vi "air.vi"() -> ()   [LabVIEW 2018]
panel:
  in  "Numeric":dbl
  in  "Numeric 2":dbl
  out "String 2":string
  out "String":string
  out "fan":dbl(slide) scale=0.0..10.0
  in  "stop 2":bool
  in  "temp-":bool
  in  "temp+":bool
  in  "stop":bool
  out "temp":dbl
  out "7 2":bool
  out "6 2":bool
  out "5 2":bool
  out "4 2":bool
  out "3 2":bool
  out "2 2":bool
  out "1 2":bool
  out "7":bool
  out "6":bool
  out "5":bool
  out "4":bool
  out "3":bool
  out "2":bool
  out "1":bool
  in  "TIMER":bool
  in  "Bio sleep":bool
  in  "Auto clean":bool
  in  "Turbo":bool
  in  "Mode":bool
  in  "swing":bool
  in  "on/off":bool
  in  "fan-":bool
  in  "fan+":bool
  # "TEMP"
  # "FAN"
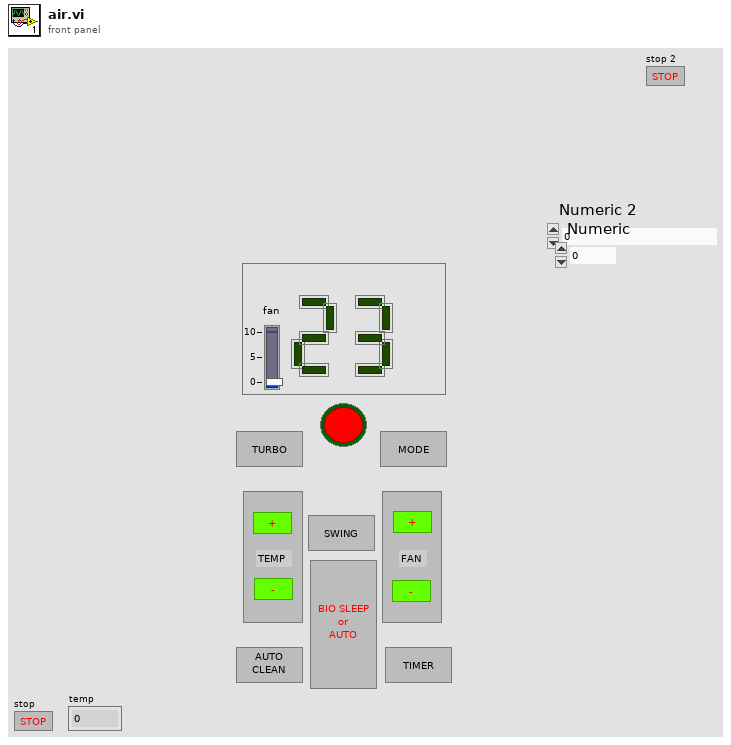
[diagram p1: front panel]
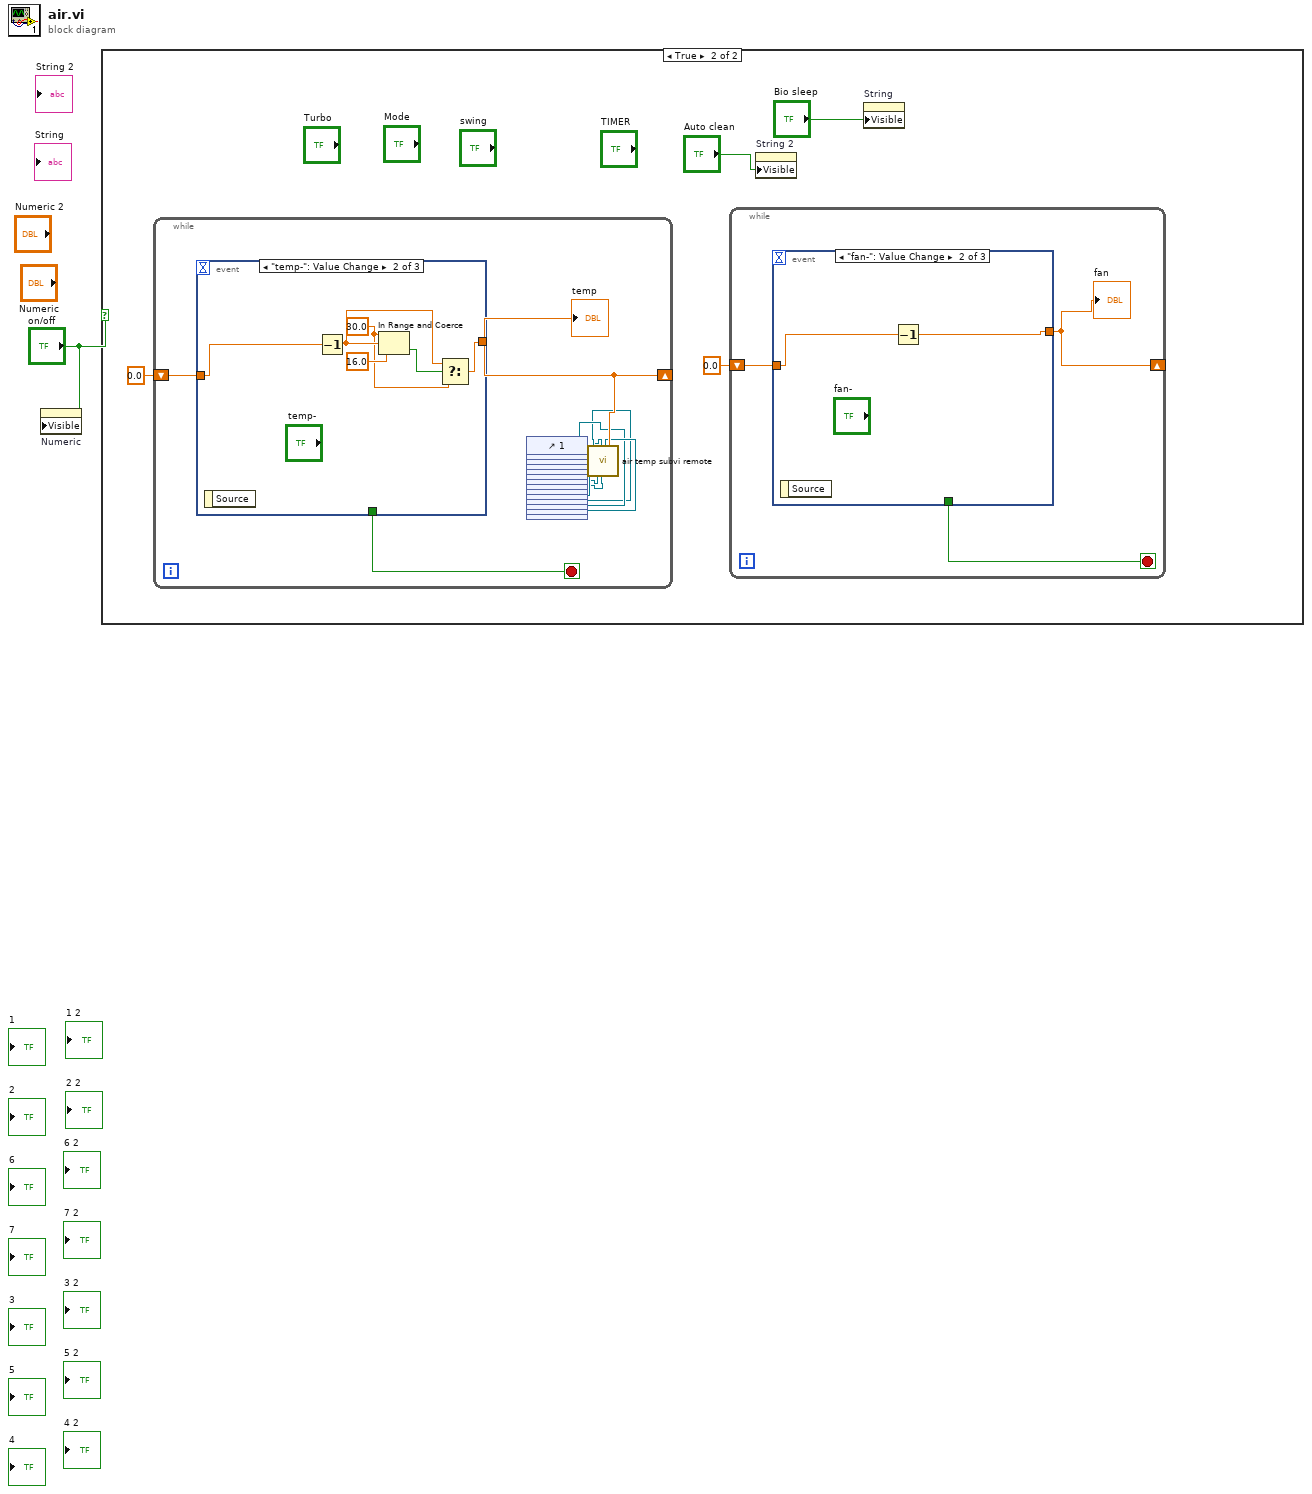
[diagram p0: block diagram]
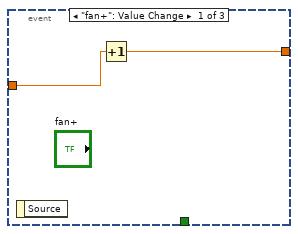
[diagram p3: hidden frame]
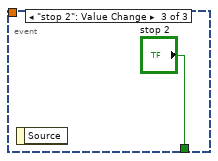
[diagram p4: hidden frame]
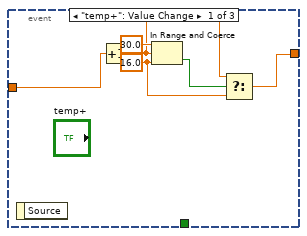
[diagram p5: hidden frame]
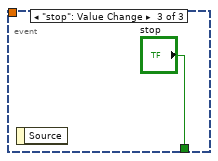
[diagram p6: hidden frame]
diagram:
  n1 = property on="Numeric" class="DigNum (strict)"("Visible"="on/off") -> ()  [unwired: 2 in, 2 out]
  n2 = case shown="True" "on/off" {
    frame False {
    }
    frame True {
      n3 = while {
        shift-right: [w28] -> _
        shift-left: 0.0 -> [w30]
        stop <- w29 stop-if-true
        n4 = event shown="[1] \"temp-\": Value Change" {
          selector: _ -> [_ _ _]
          dyn-events: _ -> [_ _ _]
          timeout: _ -> [_ _ _]
          tunnel: [w35 w37 _] -> w28
          tunnel: w30 -> [w36 w42 _]
          tunnel: [_ _ "stop"] -> w29
          event "temp+": Value Change {
            w31 = 16.0 ("lower limit")
            n5 = event-data() -> ()  [unwired: 1 in, 1 out]
            n6 = Increment(x=w36) -> (x+1=w32:dbl)
            n7 = In Range and Coerce(upper limit=30.0, x=w32, lower limit=w31) -> (In Range?=w33:bool)  [unwired: 1 out]
            n8 = Select(t=w32, s=w33, f=w31) -> (s? t:f=w35:dbl)
          }
          event "temp-": Value Change {
            w38 = 30.0 ("upper limit")
            n9 = event-data() -> ()  [unwired: 1 in, 1 out]
            n10 = Decrement(x=w42) -> (x-1=w39:dbl)
            n11 = In Range and Coerce(upper limit=w38, x=w39, lower limit=16.0) -> (In Range?=w41:bool)  [unwired: 1 out]
            n12 = Select(t=w39, s=w41, f=w38) -> (s? t:f=w37:dbl)
          }
          event "stop": Value Change {
            n13 = event-data() -> ()  [unwired: 1 in, 1 out]
          }
        }
        "temp" <- w28
        n14 = control-ref of="1"() -> (w14:refnum<vi>)
        n15 = control-ref of="2"() -> (w15:refnum<vi>)
        n16 = control-ref of="3"() -> (w16:refnum<vi>)
        n17 = control-ref of="4"() -> (w17:refnum<vi>)
        n18 = control-ref of="5"() -> (w18:refnum<vi>)
        n19 = control-ref of="6"() -> (w19:refnum<vi>)
        n20 = control-ref of="7"() -> (w20:refnum<vi>)
        n21 = control-ref of="1 2"() -> (w21:refnum<vi>)
        n22 = control-ref of="2 2"() -> (w22:refnum<vi>)
        n23 = control-ref of="3 2"() -> (w23:refnum<vi>)
        n24 = control-ref of="4 2"() -> (w24:refnum<vi>)
        n25 = control-ref of="5 2"() -> (w25:refnum<vi>)
        n26 = control-ref of="6 2"() -> (w26:refnum<vi>)
        n27 = control-ref of="7 2"() -> (w27:refnum<vi>)
        n28 = call "air temp subvi remote.vi"("Boolean in"=w26, "reference 3"=w16, "reference 11"=w24, "reference 4"=w17, "reference 10"=w23, "reference 5"=w18, "reference 6"=w19, "reference 12"=w25, "reference 7"=w20, "reference 2"=w15, "reference 8"=w21, "reference"=w14, "reference 9"=w22, "reference 14"=w27, "Numeric"=w28) -> ()  [unwired: 13 in]
      }
      n29 = while {
        shift-right: [w6] -> _
        shift-left: 0.0 -> [w8]
        stop <- w7 stop-if-true
        n30 = event shown="[1] \"fan-\": Value Change" {
          selector: _ -> [_ _ _]
          dyn-events: _ -> [_ _ _]
          timeout: _ -> [_ _ _]
          tunnel: [w10 w11 _] -> w6
          tunnel: w8 -> [w9 w12 _]
          tunnel: [_ _ "stop 2"] -> w7
          event "fan+": Value Change {
            n31 = event-data() -> ()  [unwired: 1 in, 1 out]
            n32 = Increment(x=w9) -> (x+1=w10:dbl)
          }
          event "fan-": Value Change {
            n33 = event-data() -> ()  [unwired: 1 in, 1 out]
            n34 = Decrement(x=w12) -> (x-1=w11:dbl)
          }
          event "stop 2": Value Change {
            n35 = event-data() -> ()  [unwired: 1 in, 1 out]
          }
        }
        "fan" <- w6
      }
      n36 = property on="String 2" class="Str"("Visible"="Auto clean") -> ()  [unwired: 2 in, 2 out]
      n37 = property on="String" class="Str"("Visible"="Bio sleep") -> ()  [unwired: 2 in, 2 out]
    }
  }
